vi "test Diff Configuration (Modify Add Remove).vi"(8 "error in":errorcluster, 11 "TestCase in":refnum<class "Refresh.lvclass">) -> (0 "error out":errorcluster, 3 "TestCase out":refnum<class "Refresh.lvclass">)   [LabVIEW 2020, in "Refresh.lvclass"]
uses:
  Refresh.lvclass
  Shared/1553 Channel.ctl
  Shared/Address.ctl
  Shared/Message Definition.ctl
  Shared/Message Type.ctl
  Shared/Terminal Endpoint.ctl
  Shared/Parameter Definition.ctl
  System Explorer/Implementation/System Explorer/Refresh/MCL Row.ctl
  System Explorer/Implementation/System Explorer/Refresh/Change Type.ctl
  System Explorer/Implementation/System Explorer/Refresh/Symbols.ctl
  <vilib>/addons/_JKI Toolkits/VI Tester/TestCase.llb/TestCase.lvclass
  System Explorer/Implementation/System Explorer/Refresh/Refresh.lvlib
  C:/Program Files (x86)/National Instruments/LabVIEW 2020/vi.lib/addons/_JKI Toolkits/VI Tester/TestCase.llb/TestCase.lvclass
panel:
  out "Multicolumn Listbox":i32(listbox)=-1
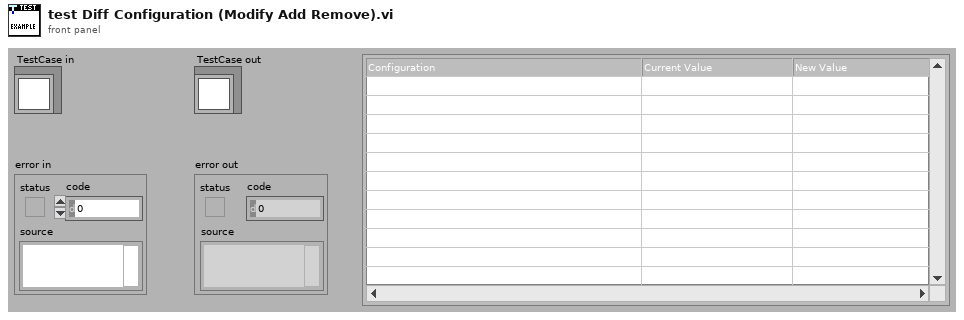
[diagram p1: front panel]
types:
  T1 = typedef "Ballard MIL-STD-1553 System Explorer.lvlib/Implementation.lvlib/Refresh.lvlib/MCL Row.ctl" = cluster{"change type":T2, "item symbol":T3, "item names":string[]}
  T2 = typedef "Ballard MIL-STD-1553 System Explorer.lvlib/Implementation.lvlib/Refresh.lvlib/Change Type.ctl" = enum16{"No change", "Modify", "Add", "Remove"}
  T3 = typedef "Ballard MIL-STD-1553 System Explorer.lvlib/Implementation.lvlib/Refresh.lvlib/Symbols.ctl" = enum16{"Blank", "MIL-STD-1553", "Port", "Remote Terminal", "Subaddress", "Bus Controller", "Acyclic Frame", "Mode Code", "Message", "Parameter", "Item"}
  T4 = typedef "1553 Channel.ctl" = cluster{"HW channel":u16, "terminal addresses":T5[], "acyclic frame names":string[], "messages":T6[]}
  T5 = typedef "Address.ctl" = u16
  T6 = typedef "Message Definition.ctl" = cluster{"name":string, "message type":T7, "endpoint Tx":T8, "endpoint Rx":T8, "create timestamp channel":bool, "mode code":u16, "number of words":u16, "parameters":cluster{"name":string, "default value":dbl, "unit":string, "parameter definition":T9}[]}
  T7 = typedef "Message Type.ctl" = string
  T8 = typedef "Terminal Endpoint.ctl" = cluster{"terminal address":T5, "subaddress":T5}
  T9 = typedef "Parameter Definition.ctl" = cluster{"start index":i32, "size (bits)":i32, "encoding":enum16{"BNR", "BCD", "Discrete"}, "signed":bool, "multiplier":dbl, "offset":dbl}
  T10 = typedef "imagedata.ctl" = cluster{"image type":i32, "image depth":i32, "image":u8[], "mask":u8[], "colors":u32[], "Rectangle":cluster{"left":i16, "top":i16, "right":i16, "bottom":i16}}
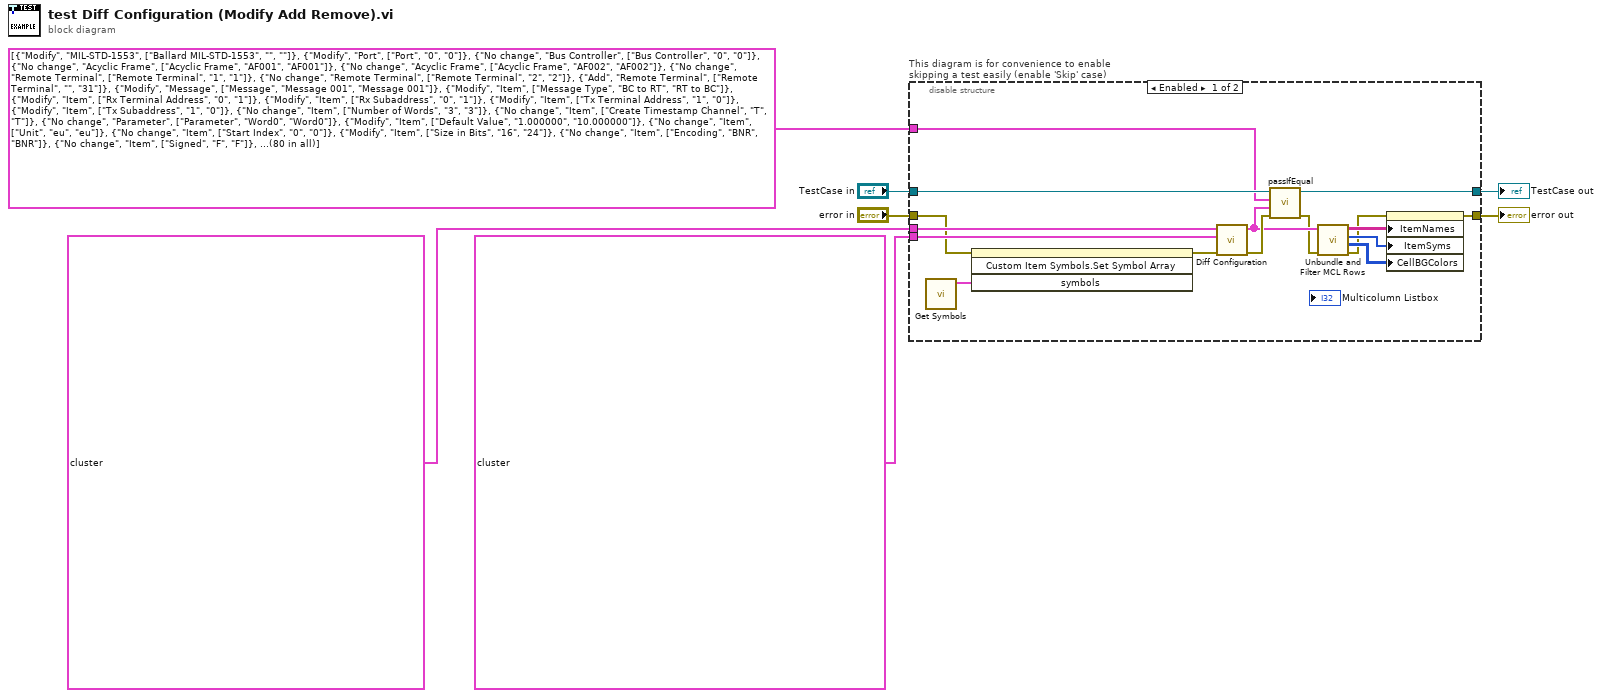
[diagram p0: block diagram]
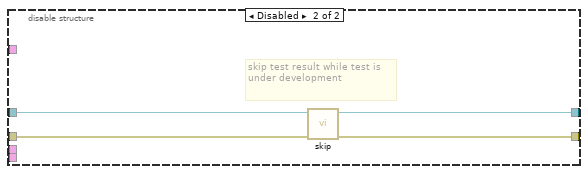
[diagram p2: hidden frame]
diagram:
  n1 = disable-structure "This diagram is for convenience to enable skipping a test easily (enable 'Skip' case)" shown="Enabled" {
    disable-tunnel: "TestCase in" -> [w23 w27]
    disable-tunnel: [w22 w25] -> w4
    disable-tunnel: [w11 w26] -> w6
    disable-tunnel: "error in" -> [w9 w24]
    disable-tunnel: T4[] [{"HW channel"=0, "terminal addresses"=[0, 1, 2], "acyclic frame names"=["AF001", "AF002"], "messages"=[{"name"="Message 001", "message type"="BC to RT", "endpoint Tx"={"terminal address"=1, "subaddress"=1}, "endpoint Rx"={"terminal address"=0, "subaddress"=0}, "create timestamp channel"=TRUE, "mode code"=0, "number of words"=3, "parameters"=[{"name"="Word0", "default value"=1.0, "unit"="eu", "parameter definition"={"start index"=0, "size (bits)"=16, "encoding"=enum."BNR", "signed"=FALSE, "multiplier"=1.0, "offset"=0.0}}, {"name"="Word1", "default value"=1.0, "unit"="eu", "parameter definition"={"start index"=16, "size (bits)"=16, "encoding"=enum."BNR", "signed"=TRUE, "multiplier"=1.0, "offset"=0.0}}, {"name"="Word2", "default value"=1.0, "unit"="eu", "parameter definition"={"start index"=32, "size (bits)"=16, "encoding"=enum."BNR", "signed"=TRUE, "multiplier"=1.0, "offset"=0.0}}]}]}, {"HW channel"=1, "terminal addresses"=[10, 11], "acyclic frame names"=[], "messages"=[{"name"="RT 10.10 to RT 11.11", "message type"="RT to RT", "endpoint Tx"={"terminal address"=10, "subaddress"=10}, "endpoint Rx"={"terminal address"=11, "subaddress"=11}, "create timestamp channel"=FALSE, "mode code"=0, "number of words"=2, "parameters"=[{"name"="P0", "default value"=1.0, "unit"="freedom units", "parameter definition"={"start index"=0, "size (bits)"=32, "encoding"=enum."BNR", "signed"=TRUE, "multiplier"=1.0, "offset"=0.0}}]}]}] ("configuration old") -> [w21 _]
    disable-tunnel: T4[] [{"HW channel"=0, "terminal addresses"=[0, 1, 2, 31], "acyclic frame names"=["AF001", "AF002"], "messages"=[{"name"="Message 001", "message type"="RT to BC", "endpoint Tx"={"terminal address"=0, "subaddress"=0}, "endpoint Rx"={"terminal address"=1, "subaddress"=1}, "create timestamp channel"=TRUE, "mode code"=0, "number of words"=3, "parameters"=[{"name"="Word0", "default value"=10.0, "unit"="eu", "parameter definition"={"start index"=0, "size (bits)"=24, "encoding"=enum."BNR", "signed"=FALSE, "multiplier"=1.0, "offset"=0.0}}, {"name"="Word1", "default value"=10.0, "unit"="eu", "parameter definition"={"start index"=24, "size (bits)"=24, "encoding"=enum."BNR", "signed"=TRUE, "multiplier"=1.0, "offset"=0.0}}]}]}, {"HW channel"=1, "terminal addresses"=[10, 11], "acyclic frame names"=[], "messages"=[{"name"="RT 10.10 to RT 11.11", "message type"="RT to RT", "endpoint Tx"={"terminal address"=10, "subaddress"=10}, "endpoint Rx"={"terminal address"=11, "subaddress"=11}, "create timestamp channel"=FALSE, "mode code"=0, "number of words"=2, "parameters"=[{"name"="P0", "default value"=1.0, "unit"="freedom units", "parameter definition"={"start index"=0, "size (bits)"=24, "encoding"=enum."BNR", "signed"=TRUE, "multiplier"=1.0, "offset"=0.0}}]}, {"name"="RT 11.21 to RT 10.20", "message type"="RT to RT", "endpoint Tx"={"terminal address"=11, "subaddress"=21}, "endpoint Rx"={"terminal address"=10, "subaddress"=20}, "create timestamp channel"=TRUE, "mode code"=0, "number of words"=0, "parameters"=[{"name"="P0", "default value"=1.0, "unit"="freedom units", "parameter definition"={"start index"=0, "size (bits)"=24, "encoding"=enum."BNR", "signed"=TRUE, "multiplier"=1.0, "offset"=0.0}}]}]}] ("configuration old") -> [w20 _]
    disable-tunnel: T1[] [{"change type"=enum."Modify", "item symbol"=enum."MIL-STD-1553", "item names"=["Ballard MIL-STD-1553", "", ""]}, {"change type"=enum."Modify", "item symbol"=enum."Port", "item names"=["Port", "0", "0"]}, {"change type"=enum."No change", "item symbol"=enum."Bus Controller", "item names"=["Bus Controller", "0", "0"]}, {"change type"=enum."No change", "item symbol"=enum."Acyclic Frame", "item names"=["Acyclic Frame", "AF001", "AF001"]}, {"change type"=enum."No change", "item symbol"=enum."Acyclic Frame", "item names"=["Acyclic Frame", "AF002", "AF002"]}, {"change type"=enum."No change", "item symbol"=enum."Remote Terminal", "item names"=["Remote Terminal", "1", "1"]}, {"change type"=enum."No change", "item symbol"=enum."Remote Terminal", "item names"=["Remote Terminal", "2", "2"]}, {"change type"=enum."Add", "item symbol"=enum."Remote Terminal", "item names"=["Remote Terminal", "", "31"]}, {"change type"=enum."Modify", "item symbol"=enum."Message", "item names"=["Message", "Message 001", "Message 001"]}, {"change type"=enum."Modify", "item symbol"=enum."Item", "item names"=["Message Type", "BC to RT", "RT to BC"]}, {"change type"=enum."Modify", "item symbol"=enum."Item", "item names"=["Rx Terminal Address", "0", "1"]}, {"change type"=enum."Modify", "item symbol"=enum."Item", "item names"=["Rx Subaddress", "0", "1"]}, {"change type"=enum."Modify", "item symbol"=enum."Item", "item names"=["Tx Terminal Address", "1", "0"]}, {"change type"=enum."Modify", "item symbol"=enum."Item", "item names"=["Tx Subaddress", "1", "0"]}, {"change type"=enum."No change", "item symbol"=enum."Item", "item names"=["Number of Words", "3", "3"]}, {"change type"=enum."No change", "item symbol"=enum."Item", "item names"=["Create Timestamp Channel", "TRUE", "TRUE"]}, {"change type"=enum."No change", "item symbol"=enum."Parameter", "item names"=["Parameter", "Word0", "Word0"]}, {"change type"=enum."Modify", "item symbol"=enum."Item", "item names"=["Default Value", "1.000000", "10.000000"]}, {"change type"=enum."No change", "item symbol"=enum."Item", "item names"=["Unit", "eu", "eu"]}, {"change type"=enum."No change", "item symbol"=enum."Item", "item names"=["Start Index", "0", "0"]}, {"change type"=enum."Modify", "item symbol"=enum."Item", "item names"=["Size in Bits", "16", "24"]}, {"change type"=enum."No change", "item symbol"=enum."Item", "item names"=["Encoding", "BNR", "BNR"]}, {"change type"=enum."No change", "item symbol"=enum."Item", "item names"=["Signed", "FALSE", "FALSE"]}, {"change type"=enum."No change", "item symbol"=enum."Item", "item names"=["Scale Multiplier", "1.000000", "1.000000"]}, {"change type"=enum."No change", "item symbol"=enum."Item", "item names"=["Scale Offset", "0.000000", "0.000000"]}, {"change type"=enum."No change", "item symbol"=enum."Parameter", "item names"=["Parameter", "Word1", "Word1"]}, {"change type"=enum."Modify", "item symbol"=enum."Item", "item names"=["Default Value", "1.000000", "10.000000"]}, {"change type"=enum."No change", "item symbol"=enum."Item", "item names"=["Unit", "eu", "eu"]}, {"change type"=enum."Modify", "item symbol"=enum."Item", "item names"=["Start Index", "16", "24"]}, {"change type"=enum."Modify", "item symbol"=enum."Item", "item names"=["Size in Bits", "16", "24"]}, {"change type"=enum."No change", "item symbol"=enum."Item", "item names"=["Encoding", "BNR", "BNR"]}, {"change type"=enum."No change", "item symbol"=enum."Item", "item names"=["Signed", "TRUE", "TRUE"]}, {"change type"=enum."No change", "item symbol"=enum."Item", "item names"=["Scale Multiplier", "1.000000", "1.000000"]}, {"change type"=enum."No change", "item symbol"=enum."Item", "item names"=["Scale Offset", "0.000000", "0.000000"]}, {"change type"=enum."Remove", "item symbol"=enum."Parameter", "item names"=["Parameter", "Word2", ""]}, {"change type"=enum."Remove", "item symbol"=enum."Item", "item names"=["Default Value", "1.000000", ""]}, {"change type"=enum."Remove", "item symbol"=enum."Item", "item names"=["Unit", "eu", ""]}, {"change type"=enum."Remove", "item symbol"=enum."Item", "item names"=["Start Index", "32", ""]}, {"change type"=enum."Remove", "item symbol"=enum."Item", "item names"=["Size in Bits", "16", ""]}, {"change type"=enum."Remove", "item symbol"=enum."Item", "item names"=["Encoding", "BNR", ""]}, {"change type"=enum."Remove", "item symbol"=enum."Item", "item names"=["Signed", "TRUE", ""]}, {"change type"=enum."Remove", "item symbol"=enum."Item", "item names"=["Scale Multiplier", "1.000000", ""]}, {"change type"=enum."Remove", "item symbol"=enum."Item", "item names"=["Scale Offset", "0.000000", ""]}, {"change type"=enum."Modify", "item symbol"=enum."Port", "item names"=["Port", "1", "1"]}, {"change type"=enum."No change", "item symbol"=enum."Remote Terminal", "item names"=["Remote Terminal", "10", "10"]}, {"change type"=enum."No change", "item symbol"=enum."Remote Terminal", "item names"=["Remote Terminal", "11", "11"]}, {"change type"=enum."Modify", "item symbol"=enum."Message", "item names"=["Message", "RT 10.10 to RT 11.11", "RT 10.10 to RT 11.11"]}, {"change type"=enum."No change", "item symbol"=enum."Item", "item names"=["Message Type", "RT to RT", "RT to RT"]}, {"change type"=enum."No change", "item symbol"=enum."Item", "item names"=["Rx Terminal Address", "11", "11"]}, {"change type"=enum."No change", "item symbol"=enum."Item", "item names"=["Rx Subaddress", "11", "11"]}, {"change type"=enum."No change", "item symbol"=enum."Item", "item names"=["Tx Terminal Address", "10", "10"]}, {"change type"=enum."No change", "item symbol"=enum."Item", "item names"=["Tx Subaddress", "10", "10"]}, {"change type"=enum."No change", "item symbol"=enum."Item", "item names"=["Number of Words", "2", "2"]}, {"change type"=enum."No change", "item symbol"=enum."Item", "item names"=["Create Timestamp Channel", "FALSE", "FALSE"]}, {"change type"=enum."No change", "item symbol"=enum."Parameter", "item names"=["Parameter", "P0", "P0"]}, {"change type"=enum."No change", "item symbol"=enum."Item", "item names"=["Default Value", "1.000000", "1.000000"]}, {"change type"=enum."No change", "item symbol"=enum."Item", "item names"=["Unit", "freedom units", "freedom units"]}, {"change type"=enum."No change", "item symbol"=enum."Item", "item names"=["Start Index", "0", "0"]}, {"change type"=enum."Modify", "item symbol"=enum."Item", "item names"=["Size in Bits", "32", "24"]}, {"change type"=enum."No change", "item symbol"=enum."Item", "item names"=["Encoding", "BNR", "BNR"]}, {"change type"=enum."No change", "item symbol"=enum."Item", "item names"=["Signed", "TRUE", "TRUE"]}, {"change type"=enum."No change", "item symbol"=enum."Item", "item names"=["Scale Multiplier", "1.000000", "1.000000"]}, {"change type"=enum."No change", "item symbol"=enum."Item", "item names"=["Scale Offset", "0.000000", "0.000000"]}, {"change type"=enum."Add", "item symbol"=enum."Message", "item names"=["Message", "", "RT 11.21 to RT 10.20"]}, {"change type"=enum."Add", "item symbol"=enum."Item", "item names"=["Message Type", "", "RT to RT"]}, {"change type"=enum."Add", "item symbol"=enum."Item", "item names"=["Rx Terminal Address", "", "10"]}, {"change type"=enum."Add", "item symbol"=enum."Item", "item names"=["Rx Subaddress", "", "20"]}, {"change type"=enum."Add", "item symbol"=enum."Item", "item names"=["Tx Terminal Address", "", "11"]}, {"change type"=enum."Add", "item symbol"=enum."Item", "item names"=["Tx Subaddress", "", "21"]}, {"change type"=enum."Add", "item symbol"=enum."Item", "item names"=["Number of Words", "", "0"]}, {"change type"=enum."Add", "item symbol"=enum."Item", "item names"=["Create Timestamp Channel", "", "TRUE"]}, {"change type"=enum."Add", "item symbol"=enum."Parameter", "item names"=["Parameter", "", "P0"]}, {"change type"=enum."Add", "item symbol"=enum."Item", "item names"=["Default Value", "", "1.000000"]}, {"change type"=enum."Add", "item symbol"=enum."Item", "item names"=["Unit", "", "freedom units"]}, {"change type"=enum."Add", "item symbol"=enum."Item", "item names"=["Start Index", "", "0"]}, {"change type"=enum."Add", "item symbol"=enum."Item", "item names"=["Size in Bits", "", "24"]}, {"change type"=enum."Add", "item symbol"=enum."Item", "item names"=["Encoding", "", "BNR"]}, {"change type"=enum."Add", "item symbol"=enum."Item", "item names"=["Signed", "", "TRUE"]}, {"change type"=enum."Add", "item symbol"=enum."Item", "item names"=["Scale Multiplier", "", "1.000000"]}, {"change type"=enum."Add", "item symbol"=enum."Item", "item names"=["Scale Offset", "", "0.000000"]}] ("configuration diff") -> [w19 _]
    frame Enabled {
      n2 = call "Get Symbols.vi"() -> ("MIL-STD-1553 symbols"=w10:T10[])  [unwired: 11 in]
      n3 = invoke on="Multicolumn Listbox" class="MCListbox (strict)" method="Custom Item Symbols.Set Symbol Array"(error in=w9, "symbols"=w10) -> (error out=w8:errorcluster)  [unwired: 2 in, 3 out]
      n4 = call "Diff Configuration.vi"("error in"=w8, "configuration new"=w20, "configuration old"=w21) -> ("error out"=w18:errorcluster, "configuration diff"=w17:T1[])  [unwired: 7 in]
      n5 = call-dynamic "passIfEqual.vi"("error in (no error)"=w18, "y"=w17, "x"=w19, "TestCase in"=w23) -> ("error out"=w13:errorcluster, "TestCase out"=w22:refnum<class "Refresh.lvclass">)  [unwired: 6 in]
      n6 = call "Unbundle and Filter MCL Rows.vi"("error in"=w13, "refresh items"=w17) -> ("error out"=w12:errorcluster, "background colors"=w16:u32[][], "item symbols"=w15:T3[], "item names"=w14:string[][])  [unwired: 6 in]
      n7 = property on="Multicolumn Listbox" class="MCListbox (strict)"(error in=w12, "ItemNames"=w14, "ItemSyms"=w15, "CellBGColors"=w16) -> (error out=w11:errorcluster)  [unwired: 1 in, 1 out]
    }
    frame Disabled {
      # "skip test result while test is under development"
      n8 = call <vilib>:"skip.vi"("error in (no error)"=w24, "TestCase in"=w27) -> ("error out"=w26:errorcluster, "TestCase out"=w25:refnum<class "Refresh.lvclass">)  [unwired: 8 in]
    }
  }
  "error out" <- w6
  "TestCase out" <- w4
